vi "Get all VIs in Project excluding Test Case VIs.vi"(8 "error in (no error)":errorcluster, 10 "Path":path, 11 "Coverage Analyzer in":refnum<class "Coverage Analyzer.lvclass">) -> (0 "error out":errorcluster, 2 "VIs":set{path}(c389), 3 "Coverage Analyzer out":refnum<class "Coverage Analyzer.lvclass">)   [LabVIEW 2020]
uses:
  Coverage Analyzer.lvclass
  2fa7b275-f75d-4bcf-8530-71b3ed265666.vi
  Coverage Analyzer.lvclass/Coverage Analyzer.ctl
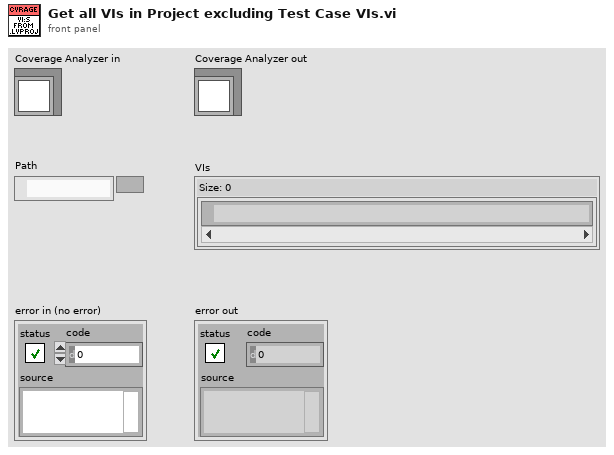
[diagram p1: front panel]
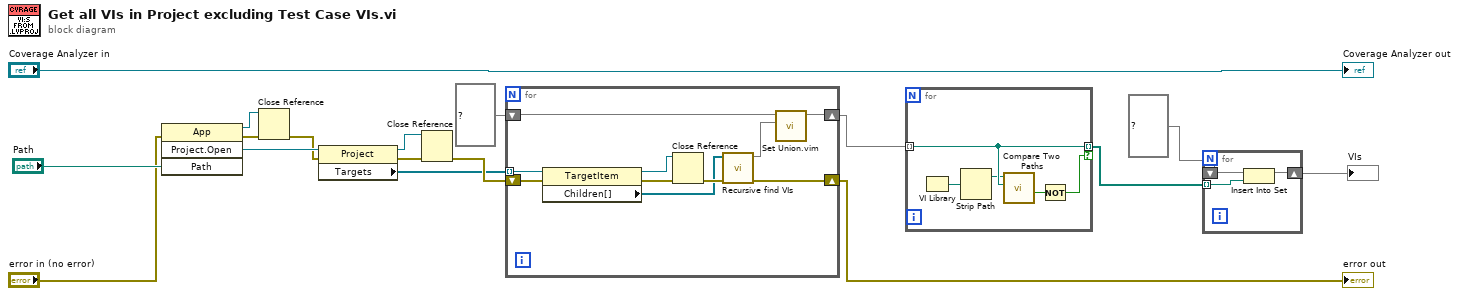
[diagram p0: block diagram]
diagram:
  n1 = invoke class="App" method="Project.Open"(error in="error in (no error)", "Path"="Path") -> (reference out=w9:refnum<vi>, error out=w14:errorcluster, "Project:Open"=w16:refnum<vi>)  [unwired: 2 in, 1 out]
  n2 = Close Reference(reference=w9, error in (no error)=w14) -> (error out=w10:errorcluster)
  n3 = property class="Project"(reference=w16, error in=w10) -> (reference out=w11:refnum<vi>, error out=w15:errorcluster, "Targets"=w1:refnum<vi>[])
  n4 = Close Reference(reference=w11, error in (no error)=w15) -> (error out=w12:errorcluster)
  n5 = for {
    tunnel: w1 -> [w27] mode=indexing
    shift-right: [w24] -> w6
    shift-left: w12 -> [w25]
    shift-right: [w20] -> w5
    shift-left: set{path} {} ("VIs") -> [w22]
    n6 = property class="TargetItem"(reference=w27, error in=w25) -> (reference out=w23:refnum<vi>, error out=w26:errorcluster, "Children[]"=w18:refnum<vi>[])
    n7 = Close Reference(reference=w23, error in (no error)=w26) -> (error out=w19:errorcluster)
    n8 = call "Recursive find VIs.vi"("error in (no error)"=w19, "Project Items"=w18) -> ("error out"=w24:errorcluster, "VIs"=w21:set{path})  [unwired: 8 in]
    n9 = call "Set Union.vim"("set 2"=w21, "set 1"=w22) -> ("union"=w20:set{path})  [unwired: 9 in]
  }
  "error out" <- w6
  n10 = for {
    tunnel: w5 -> [w29] mode=indexing
    tunnel: [w29] -> w2 mode=indexing if=w31
    n11 = VI Library() -> (path=w30:path)
    n12 = Strip Path(path=w30) -> (stripped path=w28:path)  [unwired: 1 out]
    n13 = call <vilib>:"Compare Two Paths.vi"("Path 2"=w29, "Path 1"=w28) -> ("Path 2 Relative to Path 1?"=w32:bool)  [unwired: 6 in, 3 out]
    n14 = Not(x=w32) -> (.not. x?=w31:bool)
  }
  n15 = for {
    shift-right: [w34] -> w3
    shift-left: set{path} {} ("VIs") -> [w35]
    tunnel: w2 -> [w33] mode=indexing
    n16 = Insert Into Set(10:w33, 11:w35) -> (3:w34:set{path})  [unwired: 1 out]
  }
  "VIs" <- w3
  "Coverage Analyzer out" <- "Coverage Analyzer in"
